vi "Initialize.vi"(9 "max ending temperature":dbl[unit]=273.15, 10 "starting temperature":dbl[unit]=273.15) -> (3 "Thermal Test out":refnum<class "Thermal Test.lvclass">)   [LabVIEW 2023, in "Thermal Test.lvclass"]
uses:
  Thermal Test.lvclass
  Thermal Test.lvclass/Thermal Test.ctl
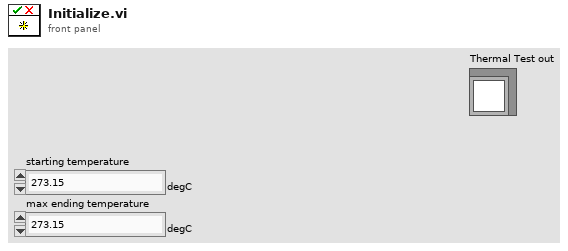
[diagram p1: front panel]
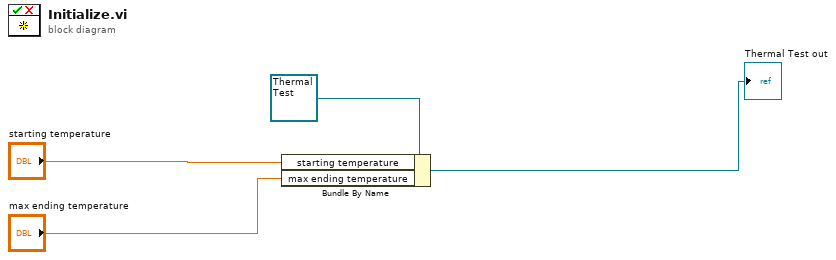
[diagram p0: block diagram]
diagram:
  n1 = Bundle By Name(cluster=refnum<class "Thermal Test.lvclass"> refnum ("Thermal Test in"), "starting temperature"="starting temperature", "max ending temperature"="max ending temperature") -> (→"Thermal Test out":refnum<class "Thermal Test.lvclass">)
